vi "Maximum Intensity_Query.vi"(1 "I(in)":dbl format="%.3f", 2 "Position for I(in)":dbl[](array[numeric]) format="%.6f", 3 "Gain for I(in)":i32=10 min=0 max=1000 step=10, 4 "Clear Maximum":bool, 5 "error in":errorcluster, 6 "I(max, in)":dbl format="%.3f", 7 "Position for I(max, in)":dbl[](array[numeric]) format="%.6f", 8 "Gain for I(max, in)":i32=10 min=0 max=1000 step=10) -> (15 "I(max, out)":dbl format="%.3f", 16 "Position for I(max, out)":dbl[](array[numeric]) format="%.6f", 17 "Gain for I(max, out)":i32=10 min=0 max=1000 step=10, 19 "error out":errorcluster)   [LabVIEW 2020]
doc: "Checks if the current intensity value (I(in)), multiplied by the current gain value (Gain for I(in)), is larger than the last maximum intensity value (I(max, in)), multiplied by the last gain value (Gain for I(max, in)), and returns the new maximum intensity values (intensity, gain and position). If Clear Maximum is TRUE, I(max, out) and Position for I(max, out) is set to zero."
panel:
  # "This vi checks if the current intensity value, multiplied by the current gain value, is larger than the\nlast maximum intensity value, multiplied by the last gain value, and returns the new maximum\nintensity values (intensity, gain and position)."
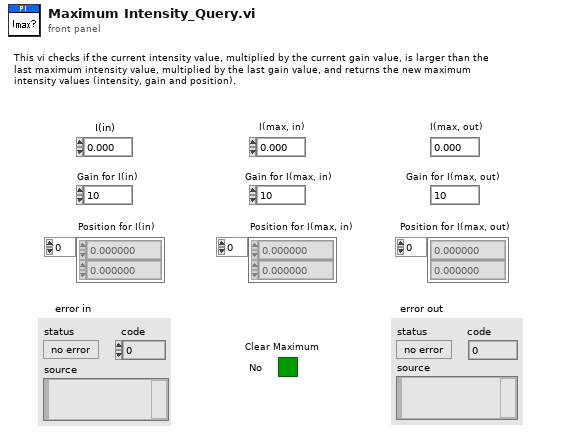
[diagram p1: front panel]
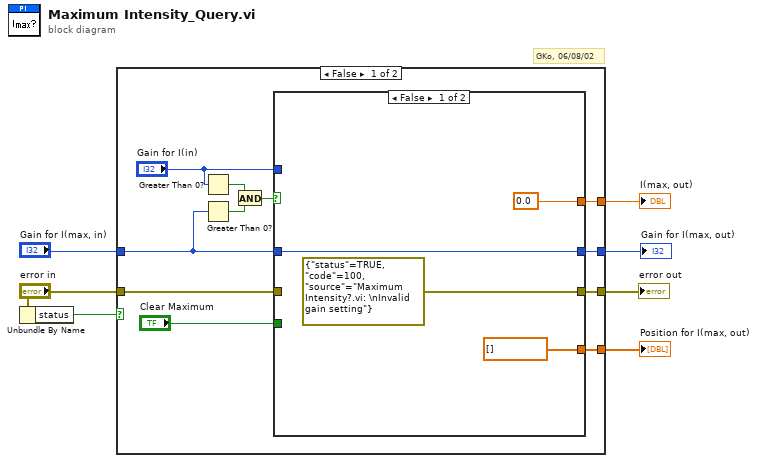
[diagram p0: block diagram]
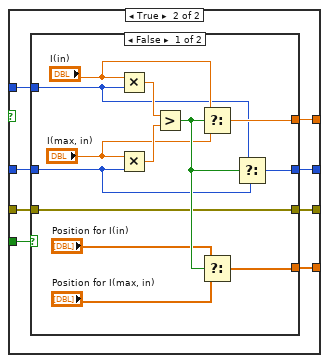
[diagram p2: hidden frame]
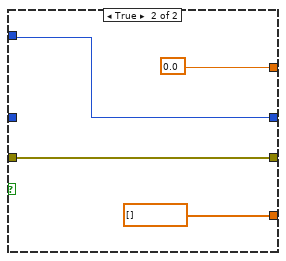
[diagram p3: hidden frame]
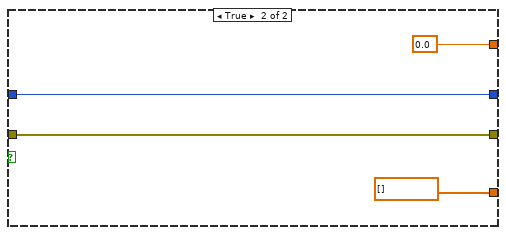
[diagram p4: hidden frame]
diagram:
  # "GKo, 06/08/02"
  n1 = Unbundle By Name("error in") -> ("status"=w7:bool)
  n2 = case shown="False" w7 {
    tunnel: "error in" -> [w14 w51]
    tunnel: [w15 w51] -> w5
    tunnel: [w12 0.0 ("I(max, out)")] -> w4
    tunnel: [w11 dbl[] [] ("Position for I(max, out)")] -> w3
    tunnel: [w10 w48] -> w2
    tunnel: "Gain for I(max, in)" -> [w8 w48]
    frame False {
      n3 = Greater Than 0?(x="Gain for I(in)") -> (x > 0?=w18:bool)
      n4 = Greater Than 0?(x=w8) -> (x > 0?=w17:bool)
      n5 = And(x=w18, y=w17) -> (x .and. y?=w16:bool)
      n6 = case shown="False" w16 {
        tunnel: [errorcluster {"status"=TRUE, "code"=100, "source"="Maximum Intensity?.vi: \nInvalid gain setting"} ("error in") w28] -> w15
        tunnel: w14 -> [_ w29]
        tunnel: "Clear Maximum" -> [_ w30]
        tunnel: [0.0 ("I(max, out)") w27] -> w12
        tunnel: [dbl[] [] ("Position for I(max, out)") w26] -> w11
        tunnel: [w19 w25] -> w10
        tunnel: w8 -> [w19 w23]
        tunnel: "Gain for I(in)" -> [_ w24]
        frame False {
        }
        frame True {
          n7 = case shown="False" w30 {
            tunnel: w29 -> [w34 w47]
            tunnel: [w34 w47] -> w28
            tunnel: [w38 0.0 ("I(max, out)")] -> w27
            tunnel: [w33 dbl[] [] ("Position for I(max, out)")] -> w26
            tunnel: [w35 w44] -> w25
            tunnel: w24 -> [w36 w44]
            tunnel: w23 -> [w37 _]
            frame False {
              n8 = Multiply(x="I(in)", y=w36) -> (x*y=w43:dbl)
              n9 = Multiply(x="I(max, in)", y=w37) -> (x*y=w42:dbl)
              n10 = Greater?(x=w43, y=w42) -> (0:w41:bool)
              n11 = Select(t="I(in)", s=w41, f="I(max, in)") -> (s? t:f=w38:dbl)
              n12 = Select(t="Position for I(in)", s=w41, f="Position for I(max, in)") -> (s? t:f=w33:dbl[])
              n13 = Select(t=w36, s=w41, f=w37) -> (s? t:f=w35:i32)
            }
            frame True {
            }
          }
        }
      }
    }
    frame True {
    }
  }
  "I(max, out)" <- w4
  "Gain for I(max, out)" <- w2
  "Position for I(max, out)" <- w3
  "error out" <- w5
